vi "Shutdown.vi"(8 "error in (no error)":errorcluster, 11 "Simulated Interlocks in":refnum<class "Simulated Interlocks.lvclass">) -> (0 "error out":errorcluster, 3 "Simulated Interlocks out":refnum<class "Simulated Interlocks.lvclass">)   [LabVIEW 2020, in "Simulated Interlocks.lvclass"]
uses:
  Simulated Interlocks.lvclass
  Simulated Interlocks.lvclass/Simulated Interlocks.ctl
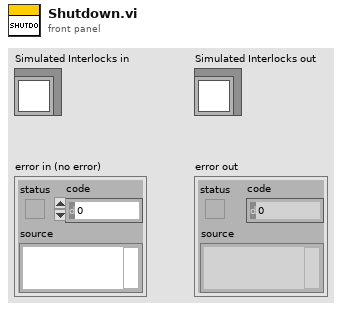
[diagram p1: front panel]
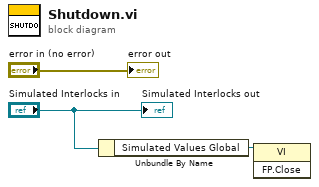
[diagram p0: block diagram]
diagram:
  n1 = Unbundle By Name("Simulated Interlocks in") -> ("Simulated Values Global"=w2:refnum<vi>)
  n2 = invoke class="VI" method="FP.Close"(reference=w2) -> ()  [unwired: 2 in, 3 out]
  "error out" <- "error in (no error)"
  "Simulated Interlocks out" <- "Simulated Interlocks in"
